vi "Read iCalendar File.vi"(8 "error in":errorcluster, 11 "Path to Open":path) -> (0 "error out":errorcluster, 1 "Extracted Data":T1, 2 "ICS String Out":string, 3 "Path Out":path)   [LabVIEW 2016]
doc: "Read iCalendar File VI opens an iCalendar file and extracts the most important information out of it."
uses:
  controls/Extract iCalendar String.ctl
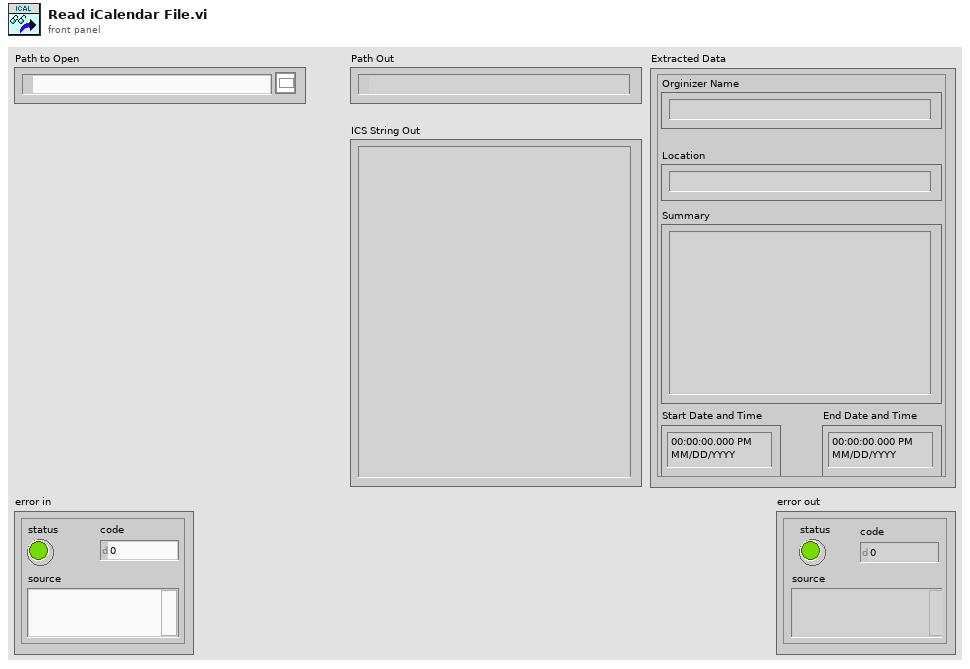
[diagram p1: front panel]
types:
  T1 = typedef "Extract iCalendar string.ctl" = cluster{"Orginizer Name":string, "Location":string, "Summary":string, "Start Date and Time":timestamp, "End Date and Time":timestamp}
  T2 = enum16{"open", "replace", "create", "open or create", "replace or create", "replace or create with confirmation"}
  T3 = cluster{"Orginizer Name":string, "Location":string, "Summary":string, "Start Date":timestamp, "End Date":timestamp}
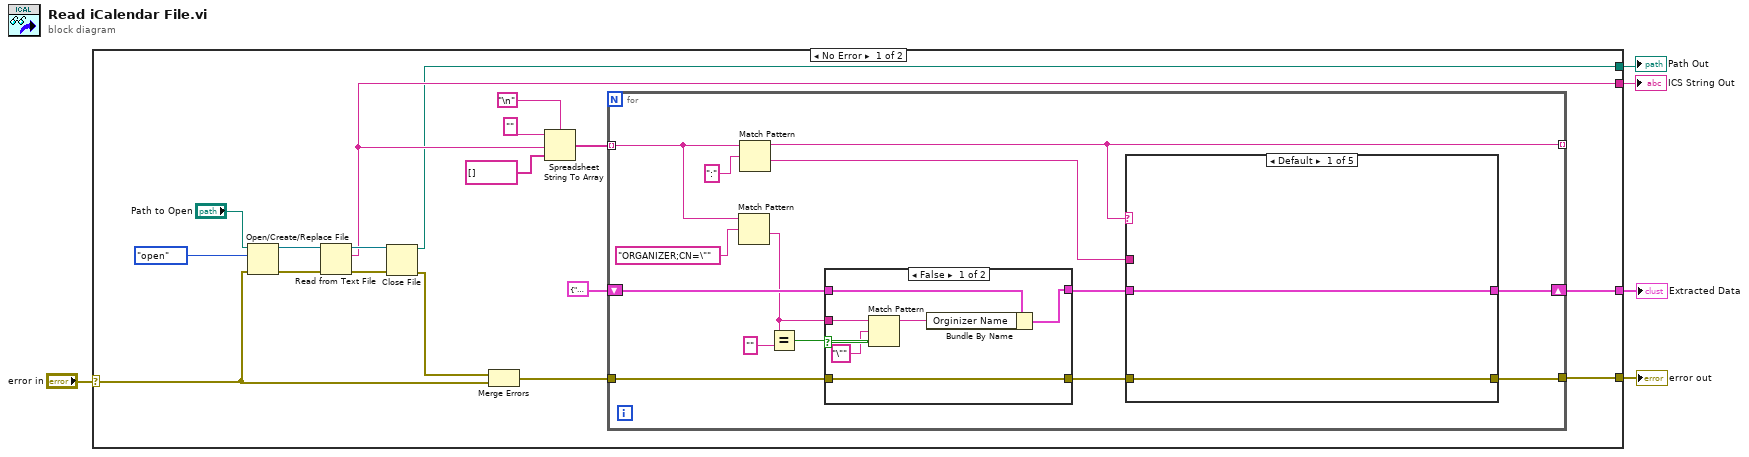
[diagram p0: block diagram]
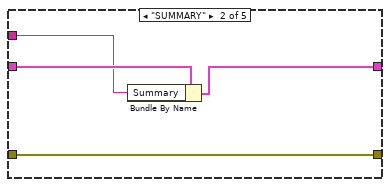
[diagram p3: hidden frame]
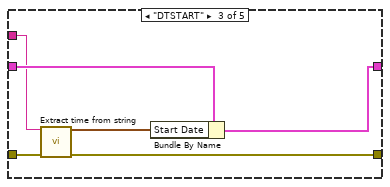
[diagram p4: hidden frame]
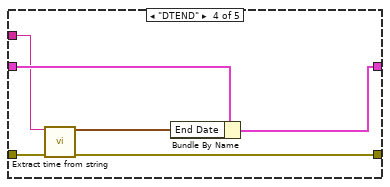
[diagram p5: hidden frame]
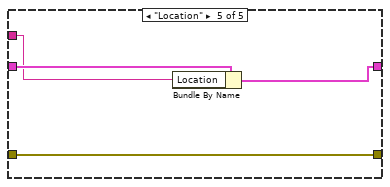
[diagram p6: hidden frame]
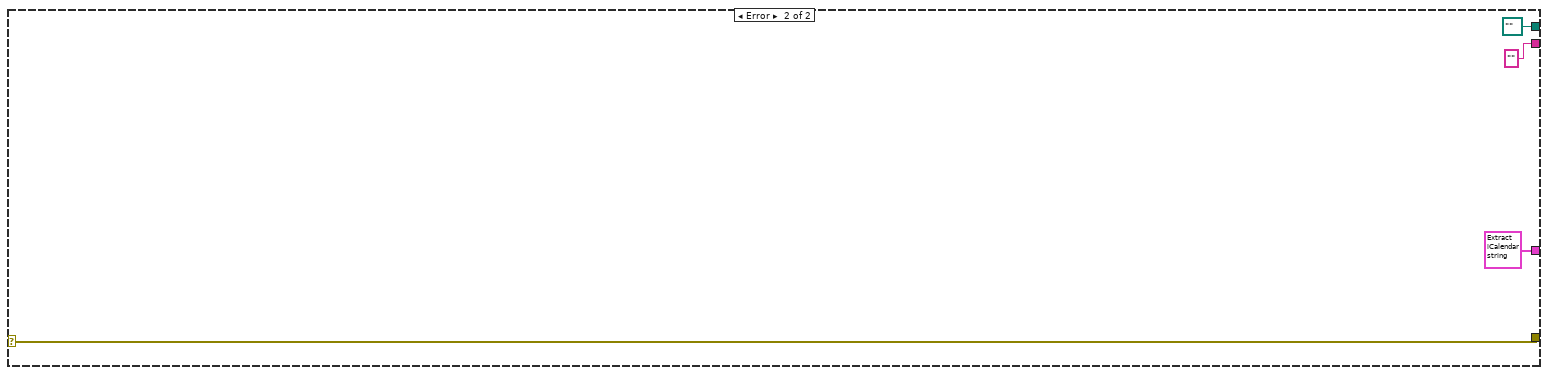
[diagram p7: hidden frame]
diagram:
  n1 = case shown="No Error" "error in" {
    selector: "error in" -> [w8 w70]
    tunnel: [w18 w70] -> w4
    tunnel: [w17 T1 {"Orginizer Name"="John", "Location"="Test location", "Summary"="John loves LabVIEW", "Start Date and Time"=timestamp(3582774000 s since 1904-01-01), "End Date and Time"=timestamp(3582777600 s since 1904-01-01)} ("Extracted data")] -> w3
    tunnel: [w10 ""] -> w2
    tunnel: [w9 path "" ("path")] -> w1
    frame No Error {
      n2 = Open/Create/Replace File(file path (use dialog)="Path to Open", error in=w8, operation (0:open)=T2."open") -> (refnum out=w13:refnum<file>, error out=w16:errorcluster)  [unwired: 3 in, 1 out]
      n3 = Read from Text File(file (use dialog)=w13, error in=w16) -> (refnum out=w14:refnum<file>, text=w10:string, error out=w15:errorcluster)  [unwired: 2 in, 1 out]
      n4 = Close File(refnum=w14, error in=w15) -> (path=w9:path, error out=w7:errorcluster)
      n5 = Merge Errors(w7, w8) -> (w6:errorcluster)
      n6 = Spreadsheet String To Array(delimiter (Tab)="\n", format string="", spreadsheet string=w10, array type (2D Dbl)=string[] []) -> (array=w20:string[])
      n7 = for {
        tunnel: w20 -> [w34] mode=indexing
        tunnel: [w37] -> _ mode=indexing
        shift-right: [w35] -> w17
        shift-left: T3 {"Orginizer Name"="", "Location"="", "Summary"="", "Start Date"=timestamp(0 s since 1904-01-01), "End Date"=timestamp(0 s since 1904-01-01)} ("output cluster") -> [w29]
        tunnel: w6 -> [w26]
        tunnel: [w24] -> w18
        n8 = Match Pattern(string=w34, regular expression="ORGANIZER;CN=\"") -> (after substring=w28:string)  [unwired: 1 in, 3 out]
        n9 = Match Pattern(string=w34, regular expression=":" ("format string")) -> (before substring=w37:string, after substring=w36:string)  [unwired: 1 in, 2 out]
        n10 = Equal?(x=w28, y="" ("format string")) -> (x = y?=w31:bool)
        n11 = case shown="False" w31 {
          tunnel: w29 -> [w43 w45]
          tunnel: w28 -> [w41 _]
          tunnel: [w42 w45] -> w27
          tunnel: w26 -> [w38 w44]
          tunnel: [w38 w44] -> w25
          frame False {
            n12 = Match Pattern(string=w41, regular expression="\"") -> (before substring=w40:string)  [unwired: 1 in, 3 out]
            n13 = Bundle By Name(cluster=w43, "Orginizer Name"=w40) -> (w42:T3)
          }
          frame True {
          }
        }
        n14 = case shown="Default" w37 {
          tunnel: w36 -> [_ w50 w55 w61 w65]
          tunnel: w27 -> [w47 w51 w57 w63 w67]
          tunnel: [w47 w49 w56 w62 w66] -> w35
          tunnel: w25 -> [w46 w48 w54 w60 w64]
          tunnel: [w46 w48 w53 w59 w64] -> w24
          frame Default {
          }
          frame "SUMMARY" {
            n15 = Bundle By Name(cluster=w51, "Summary"=w50) -> (w49:T3)
          }
          frame "DTSTART" {
            n16 = call "Extract time from string.vi"("ics time string"=w55, "Error In"=w54) -> ("Time and Date"=w52:timestamp, "Error Out"=w53:errorcluster)  [unwired: 12 in]
            n17 = Bundle By Name(cluster=w57, "Start Date"=w52) -> (w56:T3)
          }
          frame "DTEND" {
            n18 = call "Extract time from string.vi"("ics time string"=w61, "Error In"=w60) -> ("Time and Date"=w58:timestamp, "Error Out"=w59:errorcluster)  [unwired: 12 in]
            n19 = Bundle By Name(cluster=w63, "End Date"=w58) -> (w62:T3)
          }
          frame "Location" {
            n20 = Bundle By Name(cluster=w67, "Location"=w65) -> (w66:T3)
          }
        }
      }
    }
    frame Error {
    }
  }
  "error out" <- w4
  "Extracted Data" <- w3
  "ICS String Out" <- w2
  "Path Out" <- w1
